vi "niHWS Write Analog WDT.vi"(8 "error in (no error)":errorcluster, 10 "analog waveform":waveform(dbl)={"t0"=timestamp(0 s since 1904-01-01), "dt"=0.0, "Y"=[]}, 11 "waveform reference in":u32) -> (0 "error out":errorcluster, 3 "waveform reference out":u32)   [LabVIEW 2011]
doc: "Writes analog waveform data into the file beginning at the current read/write position.\n\nThis VI is only supported in LabVIEW 7.0 or later."
uses:
  niHWS Set Wfm DBL Attribute ID.ctl
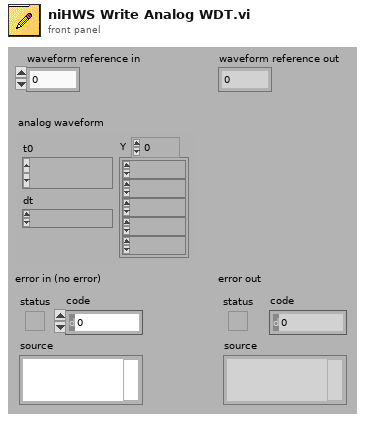
[diagram p1: front panel]
types:
  T1 = typedef "niHWS Set Wfm DBL Attribute ID.ctl" = u32
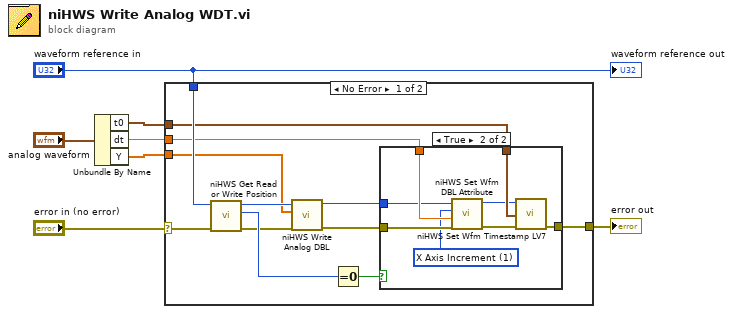
[diagram p0: block diagram]
diagram:
  n1 = Unbundle By Name("analog waveform") -> ("t0"=w3:timestamp, "dt"=w2:dbl, "Y"=w1:dbl[])
  n2 = case shown="No Error" "error in (no error)" {
    selector: "error in (no error)" -> [w17 w29]
    tunnel: [w19 w29] -> w7
    tunnel: "waveform reference in" -> [w15 _]
    tunnel: w3 -> [w10 _]
    tunnel: w2 -> [w9 _]
    tunnel: w1 -> [w8 _]
    frame No Error {
      n3 = call "niHWS Get Read or Write Position.vi"("waveform reference in"=w15, "error in (no error)"=w17) -> ("waveform reference out"=w12:u32, "position"=w16:u32, "error out"=w13:errorcluster)  [unwired: 6 in]
      n4 = call "niHWS Write Analog DBL.vi"("error in (no error)"=w13, "data"=w8, "waveform reference in"=w12) -> ("error out"=w14:errorcluster, "waveform reference out"=w11:u32)  [unwired: 7 in]
      n5 = Equal To 0?(x=w16) -> (x = 0?=w18:bool)
      n6 = case shown="True" w18 {
        tunnel: w9 -> [_ w27]
        tunnel: w10 -> [_ w26]
        tunnel: [w20 w25] -> w19
        tunnel: w14 -> [w20 w23]
        tunnel: w11 -> [_ w22]
        frame False {
        }
        frame True {
          w21 = T1 1 items=["X Axis Start"=0, "X Axis Increment"=1, "Y Axis Minimum"=3, "Y Axis Maximum"=4] ("Attribute ID")
          n7 = call "niHWS Set Wfm DBL Attribute.vi"("error in (no error)"=w23, "attribute value"=w27, "attribute ID"=w21, "waveform reference in"=w22) -> ("error out"=w28:errorcluster, "waveform reference out"=w24:u32)  [unwired: 6 in]
          n8 = call "niHWS Set Wfm Timestamp LV7.vi"("error in (no error)"=w28, "waveform timestamp"=w26, "waveform reference in"=w24) -> ("error out"=w25:errorcluster)  [unwired: 7 in, 1 out]
        }
      }
    }
    frame Error {
    }
  }
  "error out" <- w7
  "waveform reference out" <- "waveform reference in"
